vi "Add Block Diagram Content.vi"(8 "error in (no error)":errorcluster, 9 "Term Refnum":refnum<vi>, 10 "ModuleLoop":T1, 11 "FPGA Addon Input.lvclass":refnum<class "FPGA Addon Input.lvclass">) -> (0 "error out":errorcluster, 3 "FPGA Addon Input.lvclass":refnum<class "FPGA Addon Input.lvclass">)   [LabVIEW 2015, in "FPGA Addon Input.lvclass"]
uses:
  FPGA Addon Input.lvclass
  VI/VI/Module.Refs.ctl
  <vilib>/Utility/miscctls.llb/LVPointTypeDef.ctl
  <vilib>/_script/New VI Object TypeDefs/NewVIObject_LVRelativePositionTypeDef.ctl
  <vilib>/_script/New VI Object TypeDefs/NewVIObject_LVRelativeDirectionTypeDef.ctl
  <vilib>/Utility/miscctls.llb/LVPoint32TypeDef.ctl
  Signal/Read IP Core Path.vi
  Signal/Read Signal Name.vi
  VI/VI/VI.lvclass
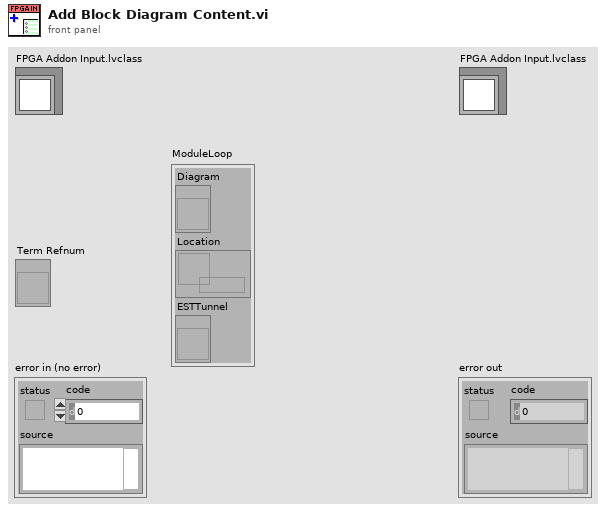
[diagram p1: front panel]
types:
  T1 = typedef "VI.lvclass/Module.Refs.ctl" = cluster{"Diagram":refnum<vi>, "Location":refnum<data-value>, "ESTTunnel":refnum<vi>}
  T2 = typedef "NewVIObject_LVRelativePositionTypeDef.ctl" = cluster{"Refnum":refnum<vi>, "Relative Direction":T3, "Point32":T4}
  T3 = typedef "NewVIObject_LVRelativeDirectionTypeDef.ctl" = enum32{"Right", "Left", "Top", "Bottom", "Top Right", "Top Left", "Bottom Right", "Bottom Left"}
  T4 = typedef "LVPoint32TypeDef.ctl" = cluster{"Horizontal":i32, "Vertical":i32}
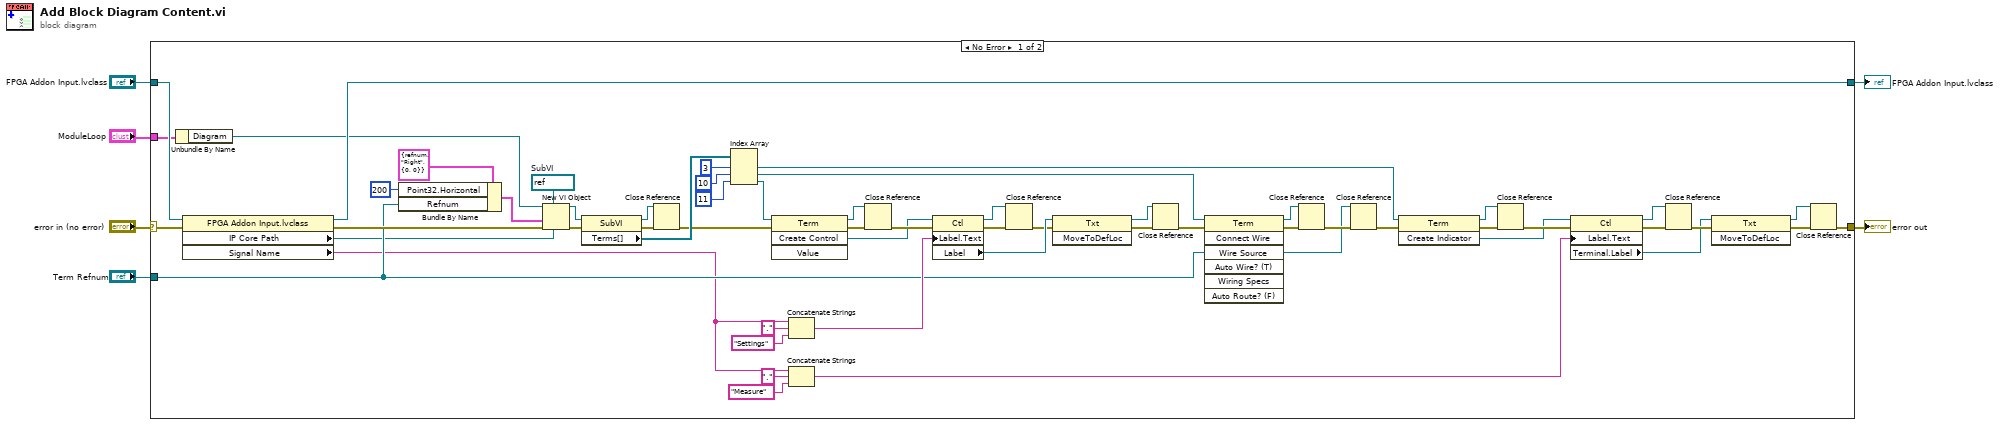
[diagram p0: block diagram]
diagram:
  n1 = case shown="No Error" "error in (no error)" {
    selector: "error in (no error)" -> [w10 w64]
    tunnel: "FPGA Addon Input.lvclass" -> [w63 w65]
    tunnel: [w62 w65] -> w5
    tunnel: "ModuleLoop" -> [w61 _]
    tunnel: [w15 w64] -> w3
    tunnel: "Term Refnum" -> [w14 _]
    frame No Error {
      w32 = refnum<vi> refnum  # SubVI
      n2 = Unbundle By Name(w61) -> ("Diagram"=w13:refnum<vi>)
      n3 = property class="FPGA Addon Input.lvclass"(reference=w63, error in=w10) -> (reference out=w62:refnum<class "FPGA Addon Input.lvclass">, error out=w16:errorcluster, "IP Core Path"=w12:path, "Signal Name"=w11:string)
      n4 = Bundle By Name(cluster=T2 {"Refnum"=refnum, "Relative Direction"=enum."Right", "Point32"={"Horizontal"=0, "Vertical"=0}} ("Relative Position"), "Point32.Horizontal"=200, "Refnum"=w14) -> (w17:T2)
      n5 = New VI Object(vi object class=w32, owner refnum=w13, position/next to=w17, 6:w12, 8:w16) -> (object refnum=w36:refnum<vi>, 0:w37:errorcluster)  [unwired: 3 in]
      n6 = property class="SubVI"(reference=w36, error in=w37) -> (reference out=w8:refnum<vi>, error out=w9:errorcluster, "Terms[]"=w33:refnum<vi>[])
      n7 = Close Reference(reference=w8, error in (no error)=w9) -> (error out=w7:errorcluster)
      n8 = Index Array(array=w33, index #1=3 ("index"), index #2=10 ("index"), index #3=11 ("index")) -> (element #1=w50:refnum<vi>, element #2=w41:refnum<vi>, element #3=w51:refnum<vi>)
      n9 = invoke class="Term" method="Create Control"(reference=w51, error in=w7) -> (reference out=w48:refnum<vi>, error out=w47:errorcluster, "Create Control"=w31:refnum<vi>)  [unwired: 2 in, 1 out]
      n10 = Concatenate Strings(w11, "." ("string"), "Settings" ("string")) -> (w38:string)
      n11 = Concatenate Strings(w11, "." ("string"), "Measure" ("string")) -> (w46:string)
      n12 = Close Reference(reference=w48, error in (no error)=w47) -> (error out=w49:errorcluster)
      n13 = property class="Ctl"(reference=w31, error in=w49, "Label.Text"=w38) -> (reference out=w30:refnum<vi>, error out=w28:errorcluster, "Label"=w29:refnum<vi>)
      n14 = Close Reference(reference=w30, error in (no error)=w28) -> (error out=w27:errorcluster)
      n15 = invoke class="Txt" method="MoveToDefLoc"(reference=w29, error in=w27) -> (reference out=w25:refnum<vi>, error out=w26:errorcluster)  [unwired: 1 in, 1 out]
      n16 = Close Reference(reference=w25, error in (no error)=w26) -> (error out=w24:errorcluster)
      n17 = invoke class="Term" method="Connect Wire"(reference=w41, error in=w24, "Wire Source"=w14) -> (reference out=w53:refnum<vi>, error out=w52:errorcluster)  [unwired: 4 in, 5 out]
      n18 = Close Reference(reference=w53, error in (no error)=w52) -> (error out=w54:errorcluster)
      n19 = Close Reference(reference=w14, error in (no error)=w54) -> (error out=w55:errorcluster)
      n20 = invoke class="Term" method="Create Indicator"(reference=w50, error in=w55) -> (reference out=w58:refnum<vi>, error out=w59:errorcluster, "Create Indicator"=w43:refnum<vi>)  [unwired: 1 in]
      n21 = Close Reference(reference=w58, error in (no error)=w59) -> (error out=w60:errorcluster)
      n22 = property class="Ctl"(reference=w43, error in=w60, "Label.Text"=w46) -> (reference out=w56:refnum<vi>, error out=w57:errorcluster, "Terminal.Label"=w21:refnum<vi>)
      n23 = Close Reference(reference=w56, error in (no error)=w57) -> (error out=w22:errorcluster)
      n24 = invoke class="Txt" method="MoveToDefLoc"(reference=w21, error in=w22) -> (reference out=w20:refnum<vi>, error out=w23:errorcluster)  [unwired: 1 in, 1 out]
      n25 = Close Reference(reference=w20, error in (no error)=w23) -> (error out=w15:errorcluster)
    }
    frame Error {
    }
  }
  "error out" <- w3
  "FPGA Addon Input.lvclass" <- w5
